vi "Drag Start Row Visualization.vi"(7 "DragStart? (F)":bool, 8 "error in (no error)":errorcluster, 10 "DragStart Indices":i32[](array[numeric]), 11 "BetterMultiListboxHandle in":refnum<class "BetterMultiListboxHandle.lvclass">) -> (0 "error out":errorcluster, 3 "BetterMultiListboxHandle out":refnum<class "BetterMultiListboxHandle.lvclass">)   [LabVIEW 2020, in "BetterDragAndDrop.lvlib" / "BetterMultiListboxHandle.lvclass"]
uses:
  BetterMultiListboxHandle.lvclass
  BetterMultiListboxHandle.lvclass/BetterMultiListboxHandle.ctl
  <vilib>/Utility/miscctls.llb/LVRowAndColumnTypeDef.ctl
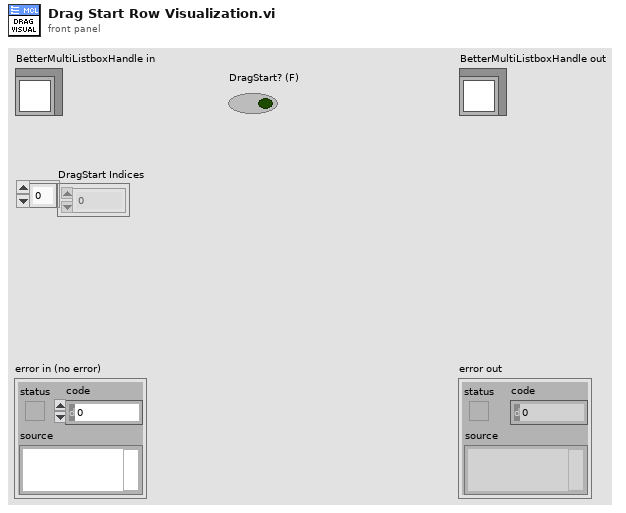
[diagram p1: front panel]
types:
  T1 = typedef "LVRowAndColumnTypeDef.ctl" = cluster{"Row":i32, "Column":i32}
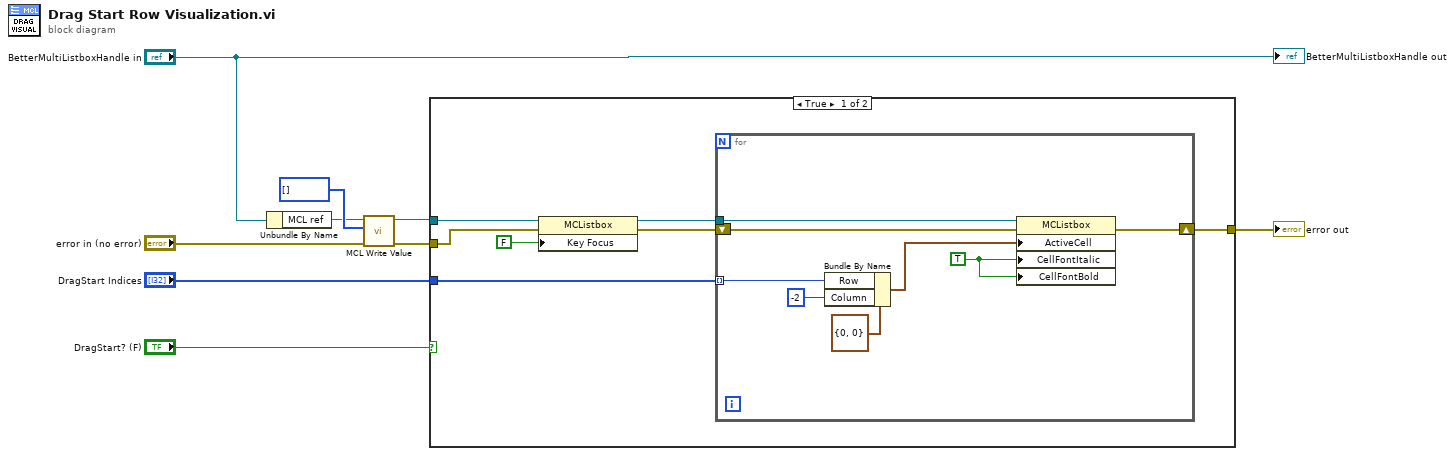
[diagram p0: block diagram]
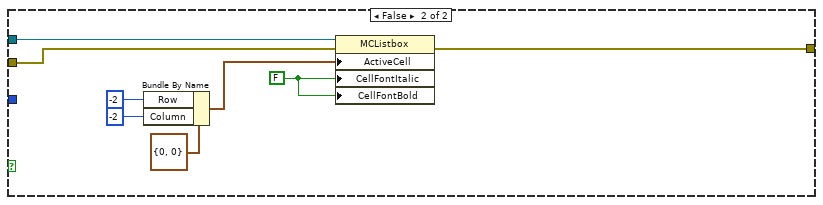
[diagram p2: hidden frame]
diagram:
  n1 = Unbundle By Name("BetterMultiListboxHandle in") -> ("MCL ref"=w5:refnum<vi>)
  n2 = call "MCL Write Value.vi"("error in (no error)"="error in (no error)", "Value"=i32[] [], "MCL Ref (generic)"=w5) -> ("error out"=w8:errorcluster, "MCL Ref (generic)"=w7:refnum<vi>)  [unwired: 7 in]
  n3 = case shown="True" "DragStart? (F)" {
    tunnel: w7 -> [w16 w27]
    tunnel: "DragStart Indices" -> [w13 _]
    tunnel: w8 -> [w11 w26]
    tunnel: [w10 w25] -> w1
    frame True {
      n4 = property class="MCListbox"(reference=w16, error in=w11, "Key Focus"=FALSE) -> (reference out=w14:refnum<vi>, error out=w12:errorcluster)
      n5 = for {
        tunnel: w14 -> [w21]
        tunnel: w13 -> [w20] mode=indexing
        shift-right: [w17] -> w10
        shift-left: w12 -> [w18]
        w19 = TRUE ("Active Cell:Cell Font:Italic")
        n6 = Bundle By Name(cluster=T1 {"Row"=0, "Column"=0} ("Active Cell:Active Cell"), "Row"=w20, "Column"=-2) -> (w22:T1)
        n7 = property class="MCListbox"(reference=w21, error in=w18, "ActiveCell"=w22, "CellFontItalic"=w19, "CellFontBold"=w19) -> (error out=w17:errorcluster)  [unwired: 1 out]
      }
    }
    frame False {
      w29 = FALSE ("Active Cell:Cell Font:Italic")
      n8 = Bundle By Name(cluster=T1 {"Row"=0, "Column"=0} ("Active Cell:Active Cell"), "Row"=-2, "Column"=-2) -> (w30:T1)
      n9 = property class="MCListbox"(reference=w27, error in=w26, "ActiveCell"=w30, "CellFontItalic"=w29, "CellFontBold"=w29) -> (error out=w25:errorcluster)  [unwired: 1 out]
    }
  }
  "error out" <- w1
  "BetterMultiListboxHandle out" <- "BetterMultiListboxHandle in"
